vi "Destructor.vi"(8 "error in":errorcluster, 11 "UserComment":refnum<class "UserComment.lvclass">) -> (0 "error out":errorcluster)   [LabVIEW 2021, in "ProligentXMLGenerator.lvlib" / "UserComment.lvclass"]
uses:
  UserComment.lvclass
  UserComment.lvclass/UserComment.ctl
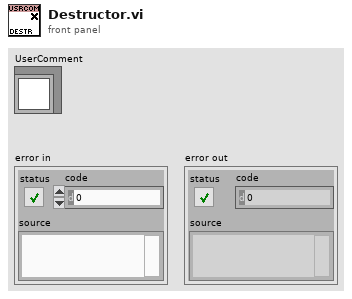
[diagram p1: front panel]
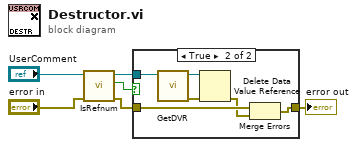
[diagram p0: block diagram]
diagram:
  n1 = call "IsRefnum.vi"("error in"="error in", "UserComment in"="UserComment") -> ("error out"=w1:errorcluster, "IsRefnum"=w3:bool, "UserComment out"=w4:refnum<class "UserComment.lvclass">)  [unwired: 7 in]
  n2 = case shown="True" w3 {
    tunnel: w1 -> [w7 w13]
    tunnel: [w7 w12] -> w6
    tunnel: w4 -> [_ w8]
    frame False {
    }
    frame True {
      n3 = call "GetDVR.vi"("UserComment"=w8) -> ("error out"=w10:errorcluster, "DVRReference"=w11:refnum<data-value>)  [unwired: 9 in]
      n4 = Delete Data Value Reference(data value reference=w11, error in=w10) -> (error out=w9:errorcluster)  [unwired: 1 out]
      n5 = Merge Errors(w13, w9) -> (w12:errorcluster)
    }
  }
  "error out" <- w6
